vi "SpreadsheetAverager.vi"() -> ()   [LabVIEW 2015]
uses:
  <vilib>/Utility/file.llb/Read Delimited Spreadsheet (DBL).vi
  <vilib>/Utility/file.llb/Write Delimited Spreadsheet (DBL).vi
panel:
  out "x/y":dbl[](array[numeric])
  in  "Number of Spreadsheets to Average":i32
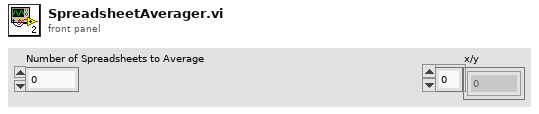
[diagram p1: front panel]
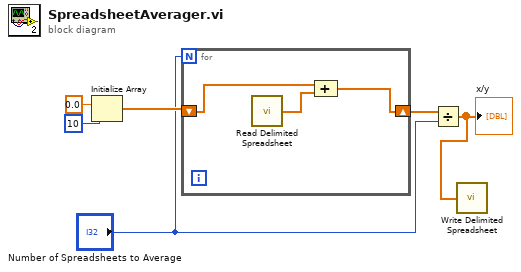
[diagram p0: block diagram]
diagram:
  n1 = Initialize Array(0.0 ("element"), 10 ("dimension size")) -> (w4:dbl[])
  n2 = for {
    N: "Number of Spreadsheets to Average" -> [_]
    shift-right: [w7] -> w3
    shift-left: w4 -> [w8]
    n3 = call-poly <vilib>:"Read Delimited Spreadsheet.vi"() -> ("first row"=w9:dbl[])  [unwired: 10 in, 5 out]
    n4 = Compound Arithmetic op=ADD(w8, w9) -> (w7:dbl[])
  }
  n5 = Divide(x=w3, y="Number of Spreadsheets to Average") -> (x/y=w1:dbl[])
  "x/y" <- w1
  n6 = call-poly <vilib>:"Write Delimited Spreadsheet.vi"("1D data"=w1) -> ()  [unwired: 13 in, 2 out]
